vi "Start Save progs.vi"(6 "table parameters":T1[](array[typedef]), 8 "error in":errorcluster, 9 "module names":string[](array[string]), 10 "messages":refnum<queue>[](array[refnum]), 11 "classes":refnum<class "Save messages PGserver.lvclass">[](array[class])) -> (0 "error out":errorcluster, 3 "size(s)":i32)   [LabVIEW 2019, in "PostgreSQL.lvlib"]
uses:
  PostgreSQL.lvlib
  Save messages PGserver/ctl/table parameters.ctl
  Save messages PGserver/Save messages PGserver.lvclass
  Save messages PGserver/Save messages PGserver.lvclass/Save messages PGserver.ctl
  Save messages PGserver/Save messages PGserver.vi
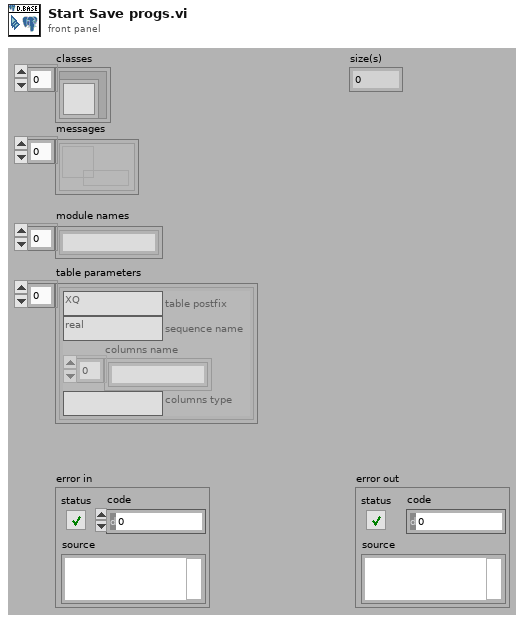
[diagram p1: front panel]
types:
  T1 = typedef "Save messages PGserver.lvclass/table parameters.ctl" = cluster{"table postfix":string, "sequence name":string, "columns name":string[], "columns type":string}
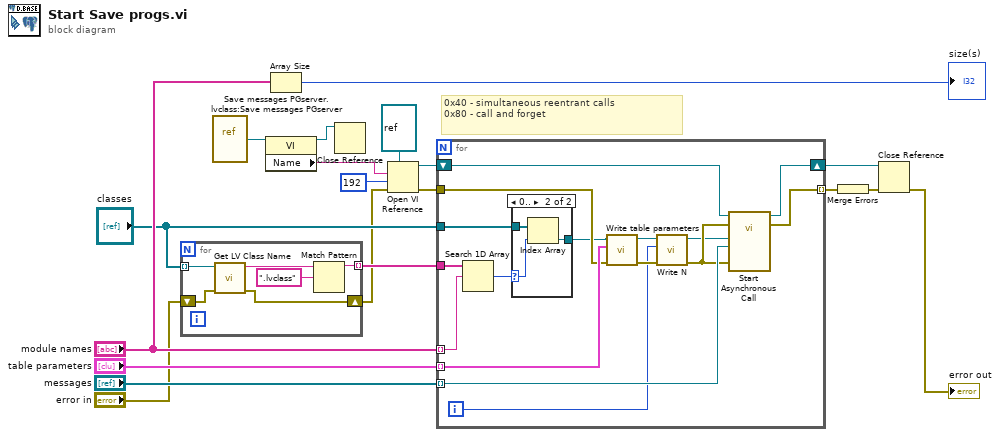
[diagram p0: block diagram]
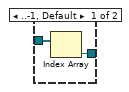
[diagram p2: hidden frame]
diagram:
  # "0x40 - simultaneous reentrant calls\n0x80 - call and forget"
  n1 = for {
    tunnel: "classes" -> [w25] mode=indexing
    tunnel: [w21] -> w4 mode=indexing
    shift-right: [w24] -> w1
    shift-left: "error in" -> [w20]
    n2 = call <vilib>:"Get LV Class Name.vi"("error in (no error)"=w20, "object"=w25) -> ("error out"=w24:errorcluster, "class name"=w23:string)  [unwired: 8 in]
    n3 = Match Pattern(string=w23, regular expression=".lvclass") -> (before substring=w21:string)  [unwired: 1 in, 3 out]
  }
  n4 = vi-ref "Save messages PGserver.lvclass:Save messages PGserver.vi"() -> (w16:refnum<vi>)
  n5 = property class="VI"(reference=w16) -> (reference out=w15:refnum<vi>, "Name"=w13:string)  [unwired: 1 in, 1 out]
  n6 = Array Size(array="module names") -> (size(s)=→"size(s)":i32)
  n7 = Close Reference(reference=w15) -> ()  [unwired: 1 in, 1 out]
  n8 = Open VI Reference(type specifier VI Refnum (for type only)=refnum<vi> refnum, vi path=w13, options=192, error in (no error)=w1) -> (vi reference=w10:refnum<vi>, error out=w12:errorcluster)  [unwired: 2 in]
  n9 = for {
    tunnel: "classes" -> [w41]
    tunnel: w4 -> [w40]
    tunnel: w12 -> [w34]
    tunnel: "table parameters" -> [w37] mode=indexing
    tunnel: "messages" -> [w36] mode=indexing
    tunnel: "module names" -> [w35] mode=indexing
    tunnel: [w32] -> w7 mode=indexing
    shift-right: [w31] -> w8
    shift-left: w10 -> [w38]
    i -> [w28]
    n10 = Search 1D Array(1D array=w40, element=w35) -> (index of element=w39:i32)  [unwired: 1 in]
    n11 = case shown="0.." w39 {
      selector: w39 -> [_ w44]
      tunnel: w41 -> [w43 w46]
      tunnel: [w42 w45] -> w33
      frame ..-1, Default {
        n12 = Index Array(array=w43) -> (element=w42:refnum<class "Save messages PGserver.lvclass">)  [unwired: 1 in]
      }
      frame 0.. {
        n13 = Index Array(array=w46, index=w44) -> (element=w45:refnum<class "Save messages PGserver.lvclass">)
      }
    }
    n14 = call "Write table parameters.vi"("error in (no error)"=w34, "table parameters"=w37, "SP in"=w33) -> ("error out"=w29:errorcluster, "SP out"=w30:refnum<class "Save messages PGserver.lvclass">)  [unwired: 7 in]
    n15 = call "Write N.vi"("error in (no error)"=w29, "N"=w28, "SP in"=w30) -> ("error out"=w27:errorcluster, "SP out"=w26:refnum<class "Save messages PGserver.lvclass">)  [unwired: 7 in]
    n16 = call-by-ref "Start Asynchronous Call"(reference=w38, error in=w27, "error in"=w27, "msg"=w36, "SP in"=w26) -> (reference out=w31:refnum<vi>, error out=w32:errorcluster)  [unwired: 6 in, 3 out]
  }
  n17 = Merge Errors(w7) -> (w6:errorcluster)
  n18 = Close Reference(reference=w8, error in (no error)=w6) -> (error out=→"error out":errorcluster)
